vi "port init.vi"(3 "error in":errorcluster, 4 "Timeout (ms)":u32=300, 5 "SerialPort":u8=1) -> (0 "error out":errorcluster, 2 "Visa Handle":refnum<visa-resource-name>)   [LabVIEW 2020]
doc: "This VI initializes RS-232 communication.\nSerial Port # COM1 = 1, COM2 = 2, etc.\nThe following parameters are fixed:\nBaud Rate = 57600; Data Bits = 8; Parity = None; Stop Bits = 1; Flow Control = XON/XOFF; Termination Character = CR/LF"
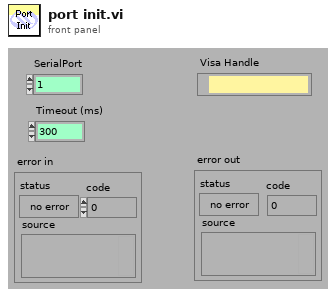
[diagram p1: front panel]
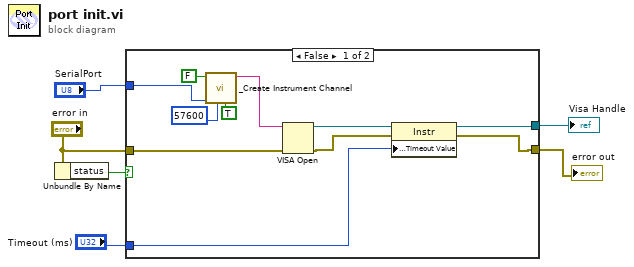
[diagram p0: block diagram]
diagram:
  n1 = Unbundle By Name("error in") -> ("status"=w6:bool)
  n2 = case shown="False" w6 {
    tunnel: "error in" -> [w13 w18]
    tunnel: [w9 w18] -> w4
    tunnel: "SerialPort" -> [w15 _]
    tunnel: [w11 _] -> w2
    tunnel: "Timeout (ms)" -> [w8 _]
    frame False {
      n3 = call "_Create Instrument Channel.vi"("XON/XOFF (False)"=TRUE, "Baud Rate (921600 - USB)"=u32 57600 ("Baud Rate (38400)"), "COM Port (1)"=w15, "(F), T - GPIB, F - RS232"=FALSE) -> ("Instrument Channel out"=w14:string)  [unwired: 5 in, 2 out]
      n4 = VISA Open(error in (no error)=w13, VISA resource name=w14) -> (VISA resource name=w12:refnum<visa-resource-name>, error out=w10:errorcluster)  [unwired: 3 in]
      n5 = property class="Instr"(reference=w12, error in=w10, "General Settings:Timeout Value"=w8) -> (reference out=w11:refnum<visa-resource-name>, error out=w9:errorcluster)
    }
    frame True {
    }
  }
  "error out" <- w4
  "Visa Handle" <- w2
